vi "SeCrTs-Alarm Ack PPSU.vi"(8 "Error in":errorcluster) -> (0 "Fehler (Ausgang)":errorcluster caption="Error out")   [LabVIEW 2022 SP3]
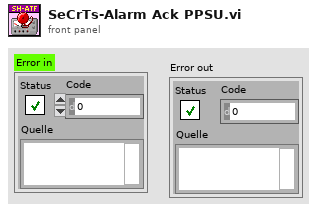
[diagram p1: front panel]
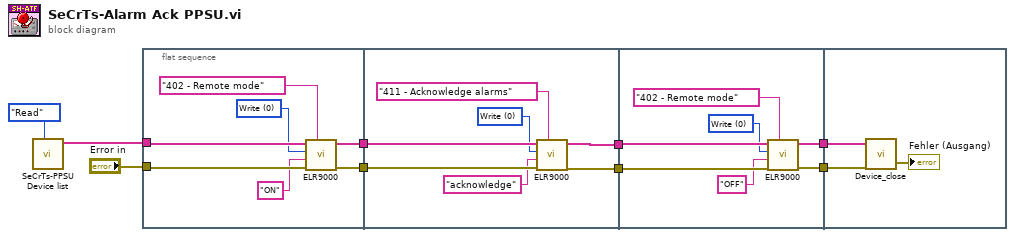
[diagram p0: block diagram]
diagram:
  n1 = call "SeCrTs-PPSU Device list.vi"("Enum"=enum16{"Read", "Write"}."Read") -> ("Device information arrayR"=w1:string[])  [unwired: 9 in, 1 out]
  n2 = flat-sequence {
    tunnel: "Error in" -> [w16]
    tunnel: w1 -> [w15]
    tunnel: [w11] -> w9
    tunnel: [w10] -> w8
    tunnel: w9 -> [w23]
    tunnel: w8 -> [w22]
    tunnel: [w18] -> w7
    tunnel: [w17] -> w6
    tunnel: w7 -> [w30]
    tunnel: w6 -> [w29]
    tunnel: [w25] -> w5
    tunnel: [w24] -> w4
    tunnel: w5 -> [w33]
    tunnel: w4 -> [w32]
    frame #0 {
      w13 = u8 0 items=["Write", "Read"] ("Access")
      n3 = call <instrlib>:"ELR9000.vi"("Command list"="402 - Remote mode", "Error in"=w16, "Value"="ON", "Access"=w13, "Device information in"=w15) -> ("Error out"=w10:errorcluster, "Device information out"=w11:string[])  [unwired: 1 in, 2 out]
    }
    frame #1 {
      w20 = u8 0 items=["Write", "Read"] ("Access")
      n4 = call <instrlib>:"ELR9000.vi"("Command list"="411 - Acknowledge alarms", "Error in"=w22, "Value"="acknowledge", "Access"=w20, "Device information in"=w23) -> ("Error out"=w18:errorcluster, "Device information out"=w17:string[])  [unwired: 1 in, 2 out]
    }
    frame #2 {
      w27 = u8 0 items=["Write", "Read"] ("Access")
      n5 = call <instrlib>:"ELR9000.vi"("Command list"="402 - Remote mode", "Error in"=w30, "Value"="OFF", "Access"=w27, "Device information in"=w29) -> ("Error out"=w25:errorcluster, "Device information out"=w24:string[])  [unwired: 1 in, 2 out]
    }
    frame #3 {
      n6 = call <instrlib>:"Device_close.vi"("error in (no error)"=w33, "Device information in"=w32) -> ("Fehler (Ausgang)"=→"Fehler (Ausgang)":errorcluster)  [unwired: 3 in]
    }
  }
